vi "CutIMG.vi"(10 "Full Image In":dbl[][](graph), 11 "Cursor List":T1) -> (2 "Cut Image Out":dbl[][](graph))   [LabVIEW 2016]
uses:
  <vilib>/Utility/miscctls.llb/LVCursorListTypeDef.ctl
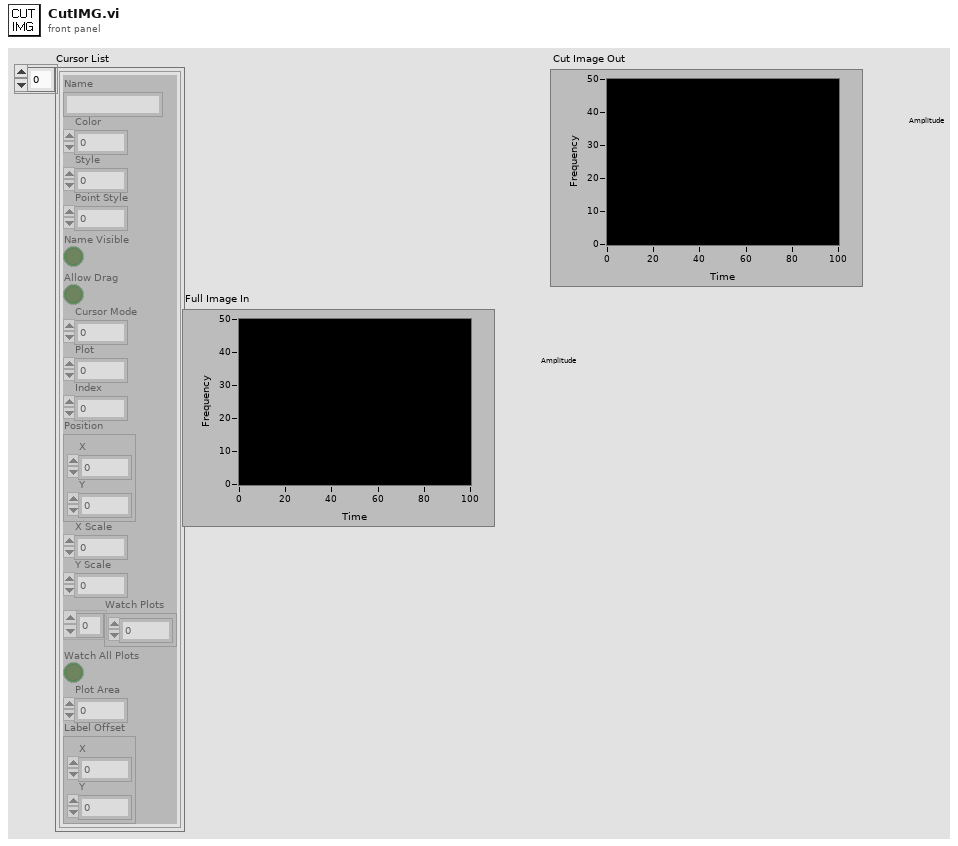
[diagram p1: front panel]
types:
  T1 = typedef "LVCursorListTypeDef.ctl" = cluster{"Name":string, "Color":u32, "Style":u8, "Point Style":u8, "Name Visible":bool, "Allow Drag":bool, "Cursor Mode":u32, "Plot":i32, "Index":i32, "Position":cluster{"X":dbl, "Y":dbl}, "X Scale":u32, "Y Scale":u32, "Watch Plots":i32[], "Watch All Plots":bool, "Plot Area":i32, "Label Offset":cluster{"X":dbl, "Y":dbl}}[]
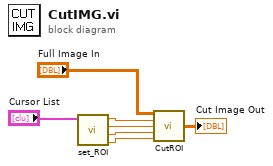
[diagram p0: block diagram]
diagram:
  n1 = call "set_ROI.vi"("Cursor List"="Cursor List") -> ("Row End"=w3:dbl, "RowStart"=w4:dbl, "ColEnd"=w5:dbl, "ColStart"=w6:dbl)  [unwired: 7 in]
  n2 = call "CutROI.vi"("Full Image In"="Full Image In", "Col Start"=w6, "Col End"=w5, "Row Start"=w4, "Row End"=w3) -> ("Cut Image Out"=→"Cut Image Out":dbl[][])  [unwired: 10 in]
